vi "Main.vi"() -> ()   [LabVIEW 2017]
doc: "This Continuous Measurement sample project is based on the Queued Message Handler template.\n\nThe Event Handling Loop generates messages based on user interface actions.\n\nThe Message Handling Loop processes messages generated by the Event Handling Loop, or by other messages. There are also Acquisition and Logging message handling loop subVIs, and a chart updating loop."
uses:
  Settings/Settings.ctl
  Acquisition/Hardware Configuration.ctl
  Acquisition/Signal Type.ctl
  Settings/Terminal Configuration.ctl
  Settings/Range.ctl
  Settings/Coupling.ctl
  Settings/Sampling Clock Source.ctl
  Settings/Time Units.ctl
  Settings/Resolution.ctl
  Settings/Trigger Direction.ctl
  Settings/Trigger Source.ctl
  Settings/Quantity.ctl
  Logging/Logging Configuration.ctl
  controls/UI Data.ctl
  controls/UI State.ctl
  support/Active channels.vi
  support/Message Queue/Enqueue Message (Single).vi
  support/Message Queue/Enqueue Message (Array).vi
  <vilib>/Utility/error.llb/Error Cluster From Error Code.vi
  <vilib>/ErrorRing/Error Ring.xnode
  Acquisition/Acquisition.lvlib
  Logging/Logging.lvlib
  Settings/Settings.lvlib
  support/User Event - Stop/User Event - Stop.lvlib
  support/Message Queue/Message Queue.lvlib
  Settings/Settings Dialog.vi
panel:
  out "Actual sampling time [s]":dbl format="%^#_6e"
  out "Ch 2":bool
  out "Ch 1":bool
  in  "Min":dbl
  in  "Max":dbl
  out "Data":waveform(dbl)[](graph)
  in  "Settings":bool
  in  "Start":bool
  in  "Stop":bool
  out "Status":string
  in  "Exit":bool
  # "Limit values"
  # "Instrumentation Idea Fast Prototyping Lab"
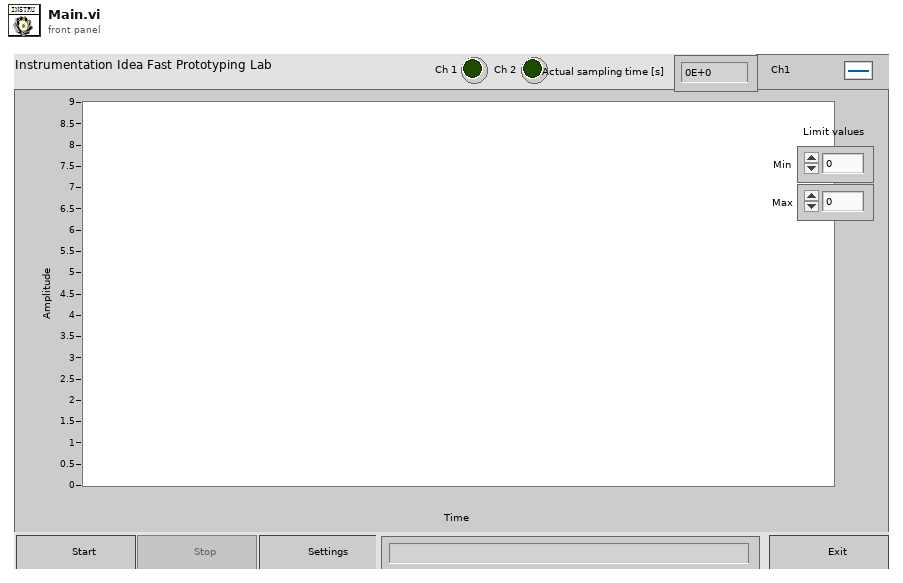
[diagram p1: front panel]
types:
  T1 = typedef "UI State.ctl" = enum16{"Idle", "Acquiring and Logging", "Waiting for Exit", "Waiting for Exit (Acq Stopped)", "Waiting for Exit (Log Stopped)", "Waiting for Stop", "Waiting for Stop (Acq Stopped)", "Waiting for Stop (Log Stopped)"}
  T2 = typedef "UI Data.ctl" = cluster{"Start Ref":refnum<vi>, "Stop Ref":refnum<vi>, "Settings Ref":refnum<vi>, "Exit Ref":refnum<vi>, "Status Ref":refnum<vi>, "Data Ref":refnum<vi>}
  T3 = typedef "Settings.lvlib/Settings.ctl" = cluster{"Hardware Configuration":T4, "Logging Configuration":T15}
  T4 = typedef "Acquisition.lvlib/Hardware Configuration.ctl" = cluster{"VISA resource name":refnum<visa-resource-name>, "DAQ Type":T5, "Channel 1":cluster{"Acquiring":bool, "Enabled":bool, "Terminal configuration":T6, "Range":T7, "Coupling":T8}, "Channel 2":cluster{"Acquiring":bool, "Enabled":bool, "Terminal configuration":T6, "Range":T7, "Coupling":T8}, "Timing":cluster{"Sample Time [Time Units]":u32, "Actual Sample Time [s]":dbl, "Samples per Iteration":u32, "Sample Clock Source":T9, "Time Units":T10, "t0":timestamp, "Baud rate":u32}, "PS Parameters":cluster{"PS handle":i16, "PS Max_adc":i16, "PS Enabled Array":i16[], "PS Device Info":cluster{"Driver Version":string, "USB Version":string, "Hardware":string, "Variant":string, "Batch and Serial":string, "Cal Date":string, "Kernel Version":string, "Digital HW Version":string, "Analogue HW Version":string, "Firmware 1":string, "Firmware 2":string, "MSO":bool, "Number of Channels":i16}, "Channel 1 Buffer":refnum<data-value>, "Channel 2 Buffer":refnum<data-value>, "Resolution":T11, "USB Power":bool}, "Trigger":cluster{"Direction":T12, "Threshold [V]":dbl, "Enabled":bool, "Trigger Source":T13}, "Keithley Parameters":cluster{"Previous End / Current Start":i32, "Quantity":T14}}
  T5 = typedef "Acquisition.lvlib/Signal Type.ctl" = u16
  T6 = typedef "Settings.lvlib/Terminal Configuration.ctl" = u16
  T7 = typedef "Settings.lvlib/Range.ctl" = u16
  T8 = typedef "Settings.lvlib/Coupling.ctl" = i16
  T9 = typedef "Settings.lvlib/Sampling Clock Source.ctl" = u16
  T10 = typedef "Settings.lvlib/Time Units.ctl" = u32
  T11 = typedef "Settings.lvlib/Resolution.ctl" = i32
  T12 = typedef "Settings.lvlib/Trigger Direction.ctl" = u16
  T13 = typedef "Settings.lvlib/Trigger Source.ctl" = u16
  T14 = typedef "Settings.lvlib/Quantity.ctl" = u16
  T15 = typedef "Logging.lvlib/Logging Configuration.ctl" = cluster{"Log File Base Path":path, "TDMS File Reference":refnum<k34>, "Enabled":bool, "Disk cache size":u64}
  T16 = typedef "Message Queue.lvlib/All Message Queues.ctl" = cluster{"UI":refnum<queue>, "Acquisition":refnum<queue>, "Logging":refnum<queue>}
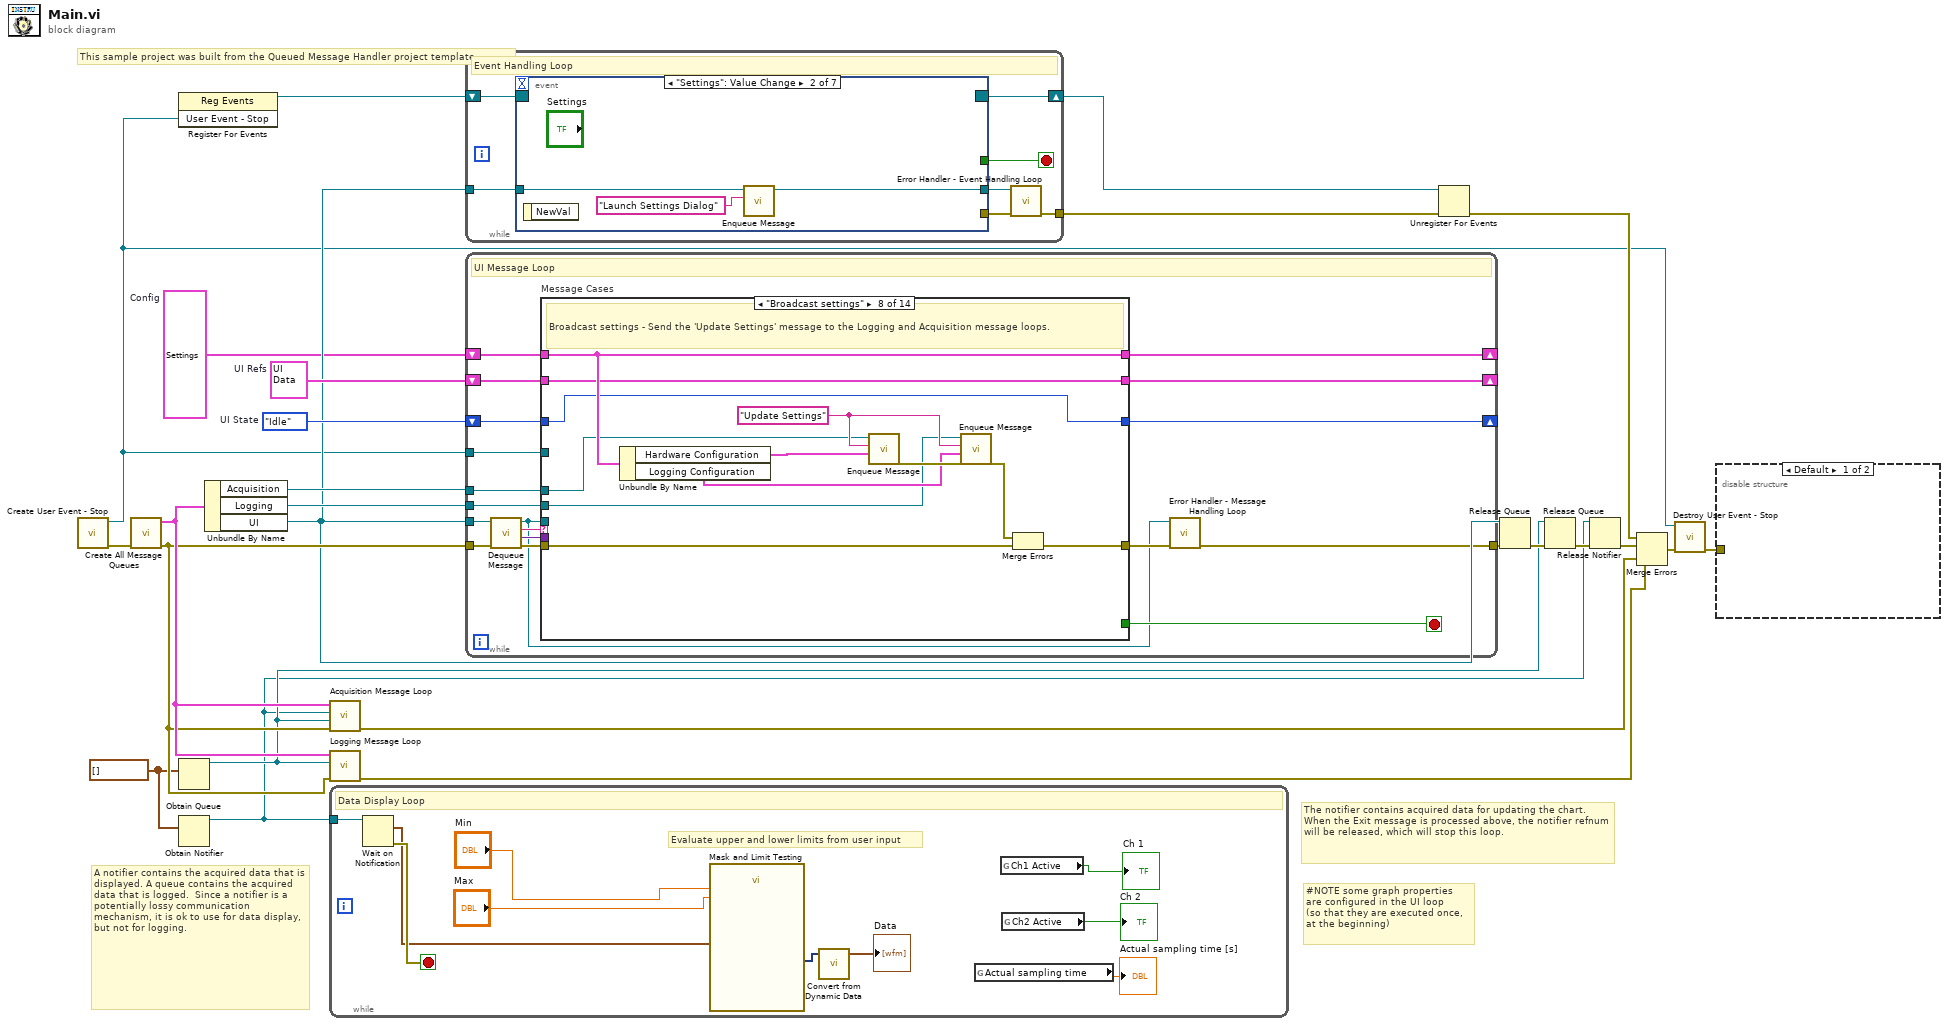
[diagram p0: block diagram]
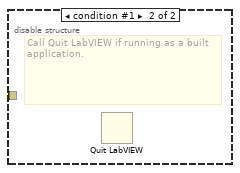
[diagram p2: hidden frame]
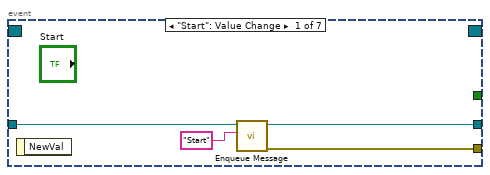
[diagram p3: hidden frame]
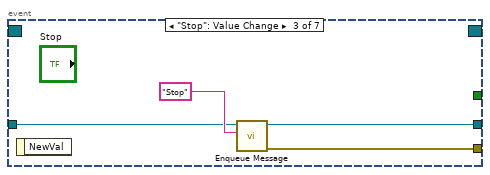
[diagram p4: hidden frame]
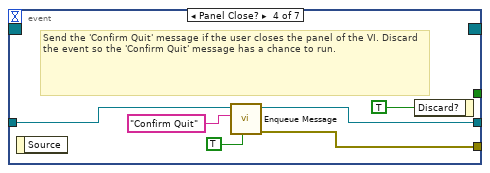
[diagram p5: hidden frame]
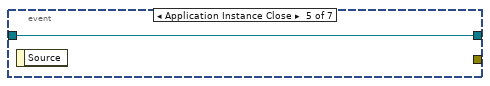
[diagram p6: hidden frame]
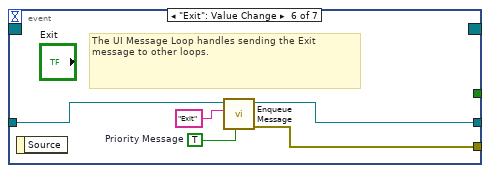
[diagram p7: hidden frame]
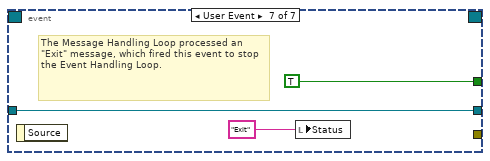
[diagram p8: hidden frame]
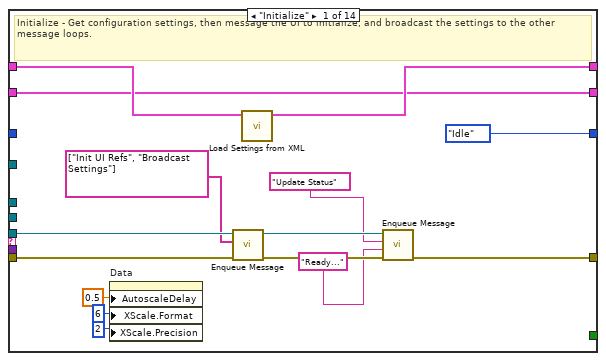
[diagram p9: hidden frame]
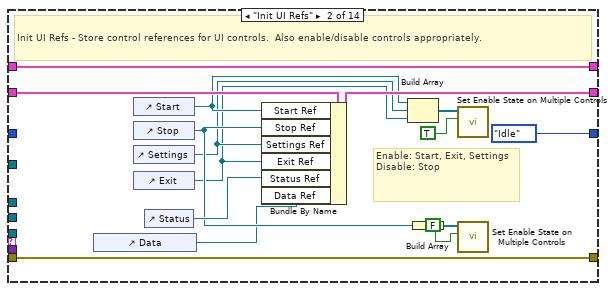
[diagram p10: hidden frame]
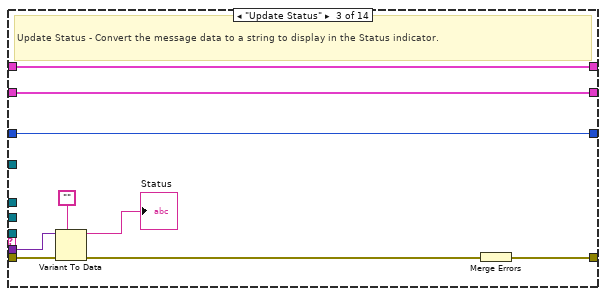
[diagram p11: hidden frame]
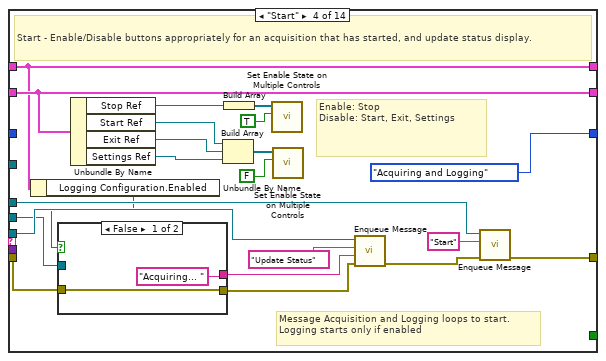
[diagram p12: hidden frame]
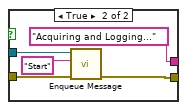
[diagram p13: hidden frame]
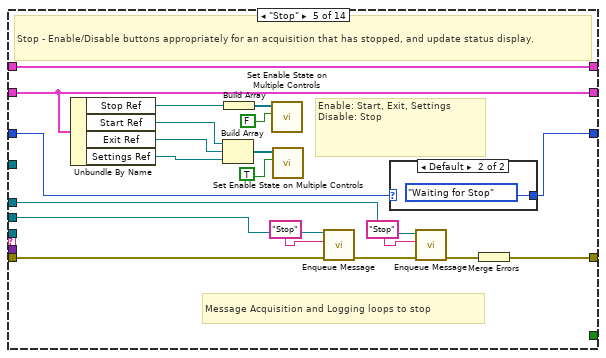
[diagram p14: hidden frame]
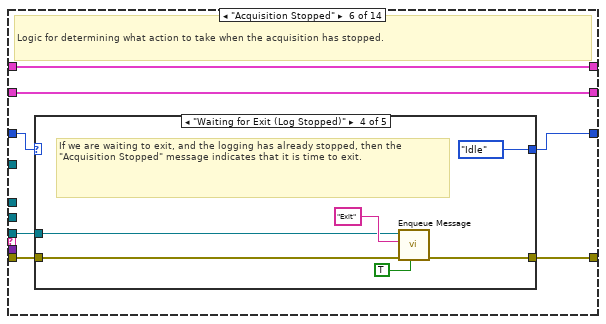
[diagram p16: hidden frame]
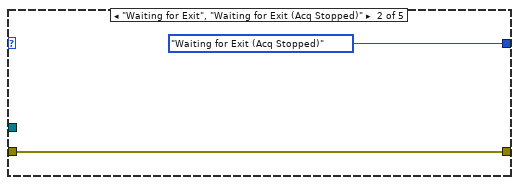
[diagram p18: hidden frame]
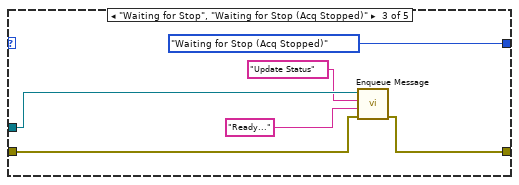
[diagram p19: hidden frame]
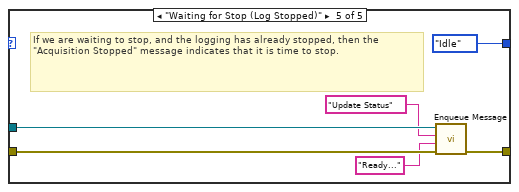
[diagram p20: hidden frame]
diagram:
  w13 = UI_State."Idle"  # UI State
  w4 = waveform(dbl)[] []
  w16 = T2 {"Start Ref"=refnum, "Stop Ref"=refnum, "Settings Ref"=refnum, "Exit Ref"=refnum, "Status Ref"=refnum, "Data Ref"=refnum}  # UI Refs
  w1 = T3 {"Hardware Configuration"={"VISA resource name"="", "DAQ Type"=0, "Channel 1"={"Acquiring"=FALSE, "Enabled"=FALSE, "Terminal configuration"=0, "Range"=32767, "Coupling"=0}, "Channel 2"={"Acquiring"=FALSE, "Enabled"=FALSE, "Terminal configuration"=0, "Range"=0, "Coupling"=0}, "Timing"={"Sample Time [Time Units]"=0, "Actual Sample Time [s]"=0.0, "Samples per Iteration"=0, "Sample Clock Source"=0, "Time Units"=0, "t0"=timestamp(0 s since 1904-01-01), "Baud rate"=0}, "PS Parameters"={"PS handle"=0, "PS Max_adc"=32767, "PS Enabled Array"=[], "PS Device Info"={"Driver Version"="", "USB Version"="", "Hardware"="", "Variant"="", "Batch and Serial"="", "Cal Date"="", "Kernel Version"="", "Digital HW Version"="", "Analogue HW Version"="", "Firmware 1"="", "Firmware 2"="", "MSO"=FALSE, "Number of Channels"=0}, "Channel 1 Buffer"=refnum, "Channel 2 Buffer"=refnum, "Resolution"=0, "USB Power"=FALSE}, "Trigger"={"Direction"=0, "Threshold [V]"=0.0, "Enabled"=FALSE, "Trigger Source"=0}, "Keithley Parameters"={"Previous End / Current Start"=0, "Quantity"=0}}, "Logging Configuration"={"Log File Base Path"=path "", "TDMS File Reference"=refnum, "Enabled"=FALSE, "Disk cache size"=0}}  # Config
  # "#NOTE some graph properties\nare configured in the UI loop \n(so that they are executed once,\nat the beginning)"
  # "This sample project was built from the Queued Message Handler project template."
  # "A notifier contains the acquired data that is displayed. A queue contains the acquired data that is logged.  Since a notifier is a potentially lossy communication mechanism, it is ok to use for data display, but not for logging."
  # "The notifier contains acquired data for updating the chart. When the Exit message is processed above, the notifier refnum will be released, which will stop this loop."
  n1 = call "Create User Event - Stop.vi"() -> ("error out"=w22:errorcluster, "User Event - Stop"=w2:refnum<user-event>)  [unwired: 10 in]
  n2 = call "Create All Message Queues.vi"("error in (no error)"=w22) -> ("error out"=w19:errorcluster, "Message Queues out"=w21:T16)  [unwired: 9 in]
  n3 = register-events(w2) -> (reference out=w3:refnum<event-registration>)  [unwired: 2 in, 1 out]
  n4 = Obtain Queue(element data type=w4) -> (queue out=w6:refnum<queue>)  [unwired: 4 in, 2 out]
  n5 = Obtain Notifier(notification data type=w4) -> (notifier out=w5:refnum<notifier>)  [unwired: 3 in, 2 out]
  n6 = Unbundle By Name(w21) -> ("Acquisition"=w15:refnum<queue>, "Logging"=w14:refnum<queue>, "UI"=w11:refnum<queue>)
  n7 = call "Acquisition Message Loop.vi"("error in (no error)"=w19, "Data Queue"=w6, "Data Notifier"=w5, "Message Queues"=w21) -> ("error out"=w23:errorcluster)  [unwired: 7 in]
  n8 = call "Logging Message Loop.vi"("error in (no error)"=w19, "Data Queue"=w6, "Message Queues"=w21) -> ("error out"=w20:errorcluster)  [unwired: 8 in]
  n9 = while "Data Display Loop" {
    tunnel: w5 -> [w35]
    stop <- w34 stop-if-true
    # "Evaluate upper and lower limits from user input"
    # "Data Display Loop"
    n10 = Wait on Notification(notifier=w35) -> (notification=w29:waveform(dbl)[], error out=w34:errorcluster)  [unwired: 3 in, 2 out]
    n11 = call "Mask and Limit Testing"("Lower Constant"="Min", "Upper Constant"="Max", "Signals"=w29) -> ("Tested Signals"=w33:dynamicdata)  [unwired: 5 in, 3 out]
    n12 = call "Convert from Dynamic Data"("Dynamic Data Type"=w33) -> ("Array of Waveform"=→"Data":waveform(dbl)[])  [unwired: 3 in]
    n13 = global read "Active channels.vi" "Actual sampling time"() -> (→"Actual sampling time [s]":dbl)
    n14 = global read "Active channels.vi" "Ch1 Active"() -> (→"Ch 1":bool)
    n15 = global read "Active channels.vi" "Ch2 Active"() -> (→"Ch 2":bool)
  }
  n16 = while {
    tunnel: w11 -> [w41]
    tunnel: [w38] -> w24
    shift-right: [w40] -> w17
    shift-left: w3 -> [w42]
    stop <- w39 stop-if-true
    # "Event Handling Loop"
    n17 = event shown="[1] \"Settings\": Value Change" {
      selector: w42 -> [_ _ _ _ _ _ _]
      dyn-events: [_ _ _ _ _ _ _] -> w40
      timeout: _ -> [_ _ _ _ _ _ _]
      tunnel: [_ _ _ _ _ _ TRUE ("Discard?")] -> w39
      tunnel: w41 -> [w46 w48 w52 w57 w60 w62 w66]
      tunnel: [w44 _ w51 w55 _ w65 _] -> w37
      tunnel: [w43 w47 w50 w56 w60 w61 w66] -> w36
      event "Start": Value Change {
        n18 = event-data() -> ()  [unwired: 1 in, 1 out]
        n19 = call-poly "Enqueue Message.vi"("Message"="Start", "Message Queue"=w46) -> ("error out"=w44:errorcluster, "dup Message Queue"=w43:refnum<queue>)  [unwired: 8 in]
      }
      event "Settings": Value Change {
        n20 = event-data() -> ()  [unwired: 1 in, 1 out]
        n21 = call-poly "Enqueue Message.vi"("Message"="Launch Settings Dialog", "Message Queue"=w48) -> ("dup Message Queue"=w47:refnum<queue>)  [unwired: 8 in, 1 out]
      }
      event "Stop": Value Change {
        n22 = event-data() -> ()  [unwired: 1 in, 1 out]
        n23 = call-poly "Enqueue Message.vi"("Message"="Stop", "Message Queue"=w52) -> ("error out"=w51:errorcluster, "dup Message Queue"=w50:refnum<queue>)  [unwired: 8 in]
      }
      event Panel Close? {
        # "Send the 'Confirm Quit' message if the user closes the panel of the VI. Discard the event so the 'Confirm Quit' message has a chance to run."
        n24 = event-data() -> ()  [unwired: 1 in, 1 out]
        n25 = call-poly "Enqueue Message.vi"("Priority Message? (F)"=TRUE, "Message"="Confirm Quit", "Message Queue"=w57) -> ("error out"=w55:errorcluster, "dup Message Queue"=w56:refnum<queue>)  [unwired: 7 in]
        n26 = event-data("Discard?"=TRUE) -> ()  [unwired: 1 in, 1 out]
      }
      event Application Instance Close {
        n27 = event-data() -> ()  [unwired: 1 in, 1 out]
      }
      event "Exit": Value Change {
        w63 = TRUE  # Priority Message
        # "The UI Message Loop handles sending the Exit message to other loops."
        n28 = event-data() -> ()  [unwired: 1 in, 1 out]
        n29 = call-poly "Enqueue Message.vi"("Priority Message? (F)"=w63, "Message"="Exit", "Message Queue"=w62) -> ("error out"=w65:errorcluster, "dup Message Queue"=w61:refnum<queue>)  [unwired: 7 in]
      }
      event User Event {
        # "The Message Handling Loop processed an \"Exit\" message, which fired this event to stop the Event Handling Loop."
        n30 = event-data() -> ()  [unwired: 1 in, 1 out]
        n31 = local write "Status"("Exit" ("Exit String")) -> ()
      }
    }
    n32 = call "Error Handler - Event Handling Loop.vi"("error in (no error)"=w37, "Message Queue"=w36) -> ("dup error in"=w38:errorcluster)  [unwired: 8 in, 1 out]
  }
  n33 = while {
    tunnel: w11 -> [w80]
    tunnel: w2 -> [w85]
    shift-right: [w70] -> _
    shift-left: w1 -> [w69]
    shift-right: [w78] -> _
    shift-left: w16 -> [w79]
    tunnel: w15 -> [w77]
    tunnel: w14 -> [w76]
    shift-right: [w71] -> _
    shift-left: w13 -> [w72]
    tunnel: w19 -> [w84]
    tunnel: [w75] -> w25
    stop <- w86 stop-if-true
    # "UI Message Loop"
    n34 = call "Dequeue Message.vi"("error in (no error)"=w84, "Message Queue"=w80) -> ("error out"=w83:errorcluster, "Message Data"=w81:variant, "Message"=w82:string, "dup Message Queue"=w73:refnum<queue>)  [unwired: 6 in]
    n35 = case "Message Cases" shown="\"Broadcast settings\"" w82 {
      selector: w82 -> [_ _ _ _ _ _ _ _ _ _ _ _ _ w316]
      tunnel: w73 -> [w93 _ _ w147 _ w179 w208 _ w248 _ w269 _ _ _]
      tunnel: w83 -> [w92 w116 w124 w129 w173 w180 w209 w236 w250 w257 w268 w297 w314 _]
      tunnel: [w97 w116 w125 w134 w174 w177 w206 w242 w243 w260 w267 w307 w313 w315] -> w74
      tunnel: [_ _ _ _ _ _ _ _ _ _ _ TRUE _ _] -> w86
      tunnel: w81 -> [_ _ w123 _ _ _ _ _ _ w261 _ w295 _ _]
      tunnel: w85 -> [_ _ _ _ _ _ _ _ _ _ _ w308 _ _]
      tunnel: [w100 w115 w119 w130 w172 w183 w212 w240 w247 w265 w272 w306 w312 w319] -> w70
      tunnel: w69 -> [w101 w115 w119 w130 w172 w183 w212 w240 w251 w265 w272 w306 w312 w319]
      tunnel: w79 -> [w94 w114 w118 w144 w171 w182 w211 w234 w245 w264 w271 w305 w311 w318]
      tunnel: [w94 w112 w118 w144 w171 w182 w211 w234 w245 w264 w271 w305 w311 w318] -> w78
      tunnel: w77 -> [_ _ _ w133 w158 _ _ w233 _ _ _ w304 _ _]
      tunnel: w76 -> [_ _ _ w135 w161 _ _ w232 _ _ _ w303 _ _]
      tunnel: w72 -> [_ _ w117 _ w155 w181 w210 w231 w244 w259 w270 _ w310 w317]
      tunnel: [UI_State."Idle" ("UI State") UI_State."Idle" ("UI State") w117 UI_State."Acquiring and Logging" ("UI State") w156 w178 w207 w231 w244 w259 w266 UI_State."Idle" ("UI State") w310 w317] -> w71
      frame "Initialize" {
        # "Initialize - Get configuration settings, then message the UI to initialize, and broadcast the settings to the other message loops."
        n36 = property on="Data" class="WFChart (strict)"("AutoscaleDelay"=sgl 0.5 ("Autoscale Delay"), "XScale.Format"=u8 6 ("X Scale.Display Format:Format"), "XScale.Precision"=u8 2 ("X Scale.Display Format:Precision")) -> ()  [unwired: 2 in, 2 out]
        n37 = call-poly "Enqueue Message.vi"("error in (no error)"=w92, "Message Array"=string[] ["Init UI Refs", "Broadcast Settings"], "Message Queue"=w93) -> ("error out"=w99:errorcluster, "dup Message Queue"=w98:refnum<queue>)  [unwired: 7 in]
        n38 = call "Load Settings from XML.vi"("Settings in"=w101) -> ("Settings out"=w100:T3)  [unwired: 9 in, 1 out]
        n39 = call-poly "Enqueue Message.vi"("error in (no error)"=w99, "Message Data"="Ready..." ("Ready..."), "Message"="Update Status", "Message Queue"=w98) -> ("error out"=w97:errorcluster)  [unwired: 6 in, 1 out]
      }
      frame "Init UI Refs" {
        # "Enable: Start, Exit, Settings\nDisable: Stop"
        # "Init UI Refs - Store control references for UI controls.  Also enable/disable controls appropriately."
        n40 = control-ref of="Data"() -> (w102:refnum<vi>)
        n41 = control-ref of="Start"() -> (w106:refnum<vi>)
        n42 = control-ref of="Stop"() -> (w107:refnum<vi>)
        n43 = control-ref of="Settings"() -> (w105:refnum<vi>)
        n44 = control-ref of="Exit"() -> (w104:refnum<vi>)
        n45 = control-ref of="Status"() -> (w113:refnum<vi>)
        n46 = Bundle By Name(cluster=w114, "Start Ref"=w106, "Stop Ref"=w107, "Settings Ref"=w105, "Exit Ref"=w104, "Status Ref"=w113, "Data Ref"=w102) -> (w112:T2)
        n47 = Build Array(w106, w105, w104) -> (w110:refnum<vi>[])
        n48 = Build Array(w107) -> (w109:refnum<vi>[])
        n49 = call "Set Enable State on Multiple Controls.vi"("Enable?"=TRUE, "Controls"=w110) -> ()  [unwired: 10 in]
        n50 = call "Set Enable State on Multiple Controls.vi"("Enable?"=FALSE, "Controls"=w109) -> ()  [unwired: 10 in]
      }
      frame "Update Status" {
        # "Update Status - Convert the message data to a string to display in the Status indicator."
        n51 = Variant To Data(error in=w124, type="", Variant=w123) -> (data=→"Status":string, error out=w121:errorcluster)
        n52 = Merge Errors(w121) -> (w125:errorcluster)
      }
      frame "Start" {
        # "Message Acquisition and Logging loops to start.\nLogging starts only if enabled"
        # "Enable: Stop\nDisable: Start, Exit, Settings"
        # "Start - Enable/Disable buttons appropriately for an acquisition that has started, and update status display."
        n53 = Unbundle By Name(w130) -> ("Logging Configuration.Enabled"=w126:bool)
        n54 = case shown="False" w126 {
          tunnel: ["Acquiring... " ("Acquiring and Logging...") "Acquiring and Logging..." ("Acquiring and Logging...")] -> w146
          tunnel: w135 -> [_ w153]
          tunnel: w129 -> [w148 w151]
          tunnel: [w148 w150] -> w128
          frame False {
          }
          frame True {
            n55 = call-poly "Enqueue Message.vi"("error in (no error)"=w151, "Message"="Start", "Message Queue"=w153) -> ("error out"=w150:errorcluster)  [unwired: 7 in, 1 out]
          }
        }
        n56 = Unbundle By Name(w144) -> ("Stop Ref"=w139:refnum<vi>, "Start Ref"=w138:refnum<vi>, "Exit Ref"=w137:refnum<vi>, "Settings Ref"=w136:refnum<vi>)
        n57 = Build Array(w138, w137, w136) -> (w142:refnum<vi>[])
        n58 = Build Array(w139) -> (w141:refnum<vi>[])
        n59 = call "Set Enable State on Multiple Controls.vi"("Enable?"=TRUE, "Controls"=w141) -> ()  [unwired: 10 in]
        n60 = call "Set Enable State on Multiple Controls.vi"("Enable?"=FALSE, "Controls"=w142) -> ()  [unwired: 10 in]
        n61 = call-poly "Enqueue Message.vi"("error in (no error)"=w128, "Message Data"=w146, "Message"="Update Status", "Message Queue"=w147) -> ("error out"=w127:errorcluster)  [unwired: 6 in, 1 out]
        n62 = call-poly "Enqueue Message.vi"("error in (no error)"=w127, "Message"="Start", "Message Queue"=w133) -> ("error out"=w134:errorcluster)  [unwired: 7 in, 1 out]
      }
      frame "Stop" {
        # "Message Acquisition and Logging loops to stop"
        # "Enable: Start, Exit, Settings\nDisable: Stop"
        # "Stop - Enable/Disable buttons appropriately for an acquisition that has stopped, and update status display."
        n63 = Unbundle By Name(w171) -> ("Stop Ref"=w166:refnum<vi>, "Start Ref"=w165:refnum<vi>, "Exit Ref"=w164:refnum<vi>, "Settings Ref"=w163:refnum<vi>)
        n64 = Build Array(w165, w164, w163) -> (w169:refnum<vi>[])
        n65 = Build Array(w166) -> (w168:refnum<vi>[])
        n66 = call "Set Enable State on Multiple Controls.vi"("Enable?"=FALSE, "Controls"=w168) -> ()  [unwired: 10 in]
        n67 = call "Set Enable State on Multiple Controls.vi"("Enable?"=TRUE, "Controls"=w169) -> ()  [unwired: 10 in]
        n68 = call-poly "Enqueue Message.vi"("error in (no error)"=w173, "Message"="Stop", "Message Queue"=w161) -> ("error out"=w160:errorcluster)  [unwired: 7 in, 1 out]
        n69 = case shown="Default" w155 {
          selector: w155 -> [w175 _]
          tunnel: [w175 UI_State."Waiting for Stop" ("UI State")] -> w156
          frame "Waiting for Exit" {
          }
          frame Default {
          }
        }
        n70 = call-poly "Enqueue Message.vi"("error in (no error)"=w160, "Message"="Stop", "Message Queue"=w158) -> ("error out"=w159:errorcluster)  [unwired: 7 in, 1 out]
        n71 = Merge Errors(w159) -> (w174:errorcluster)
      }
      frame "Acquisition Stopped" {
        # "Logic for determining what action to take when the acquisition has stopped."
        n72 = case shown="\"Waiting for Exit (Log Stopped)\"" w181 {
          selector: w181 -> [w185 _ _ _ _]
          tunnel: w180 -> [w184 w187 w189 w194 w205]
          tunnel: w179 -> [_ _ w192 w195 w202]
          tunnel: [w185 UI_State."Waiting for Exit (Acq Stopped)" ("UI State") UI_State."Waiting for Stop (Acq Stopped)" ("UI State") UI_State."Idle" ("UI State") UI_State."Idle" ("UI State")] -> w178
          tunnel: [w184 w187 w188 w199 w203] -> w177
          frame Default {
          }
          frame "Waiting for Exit", "Waiting for Exit (Acq Stopped)" {
          }
          frame "Waiting for Stop", "Waiting for Stop (Acq Stopped)" {
            n73 = call-poly "Enqueue Message.vi"("error in (no error)"=w189, "Message Data"="Ready..." ("Ready..."), "Message"="Update Status", "Message Queue"=w192) -> ("error out"=w188:errorcluster)  [unwired: 6 in, 1 out]
          }
          frame "Waiting for Exit (Log Stopped)" {
            # "If we are waiting to exit, and the logging has already stopped, then the \"Acquisition Stopped\" message indicates that it is time to exit."
            n74 = call-poly "Enqueue Message.vi"("Priority Message? (F)"=TRUE, "error in (no error)"=w194, "Message"="Exit", "Message Queue"=w195) -> ("error out"=w199:errorcluster)  [unwired: 6 in, 1 out]
          }
          frame "Waiting for Stop (Log Stopped)" {
            # "If we are waiting to stop, and the logging has already stopped, then the \"Acquisition Stopped\" message indicates that it is time to stop."
            n75 = call-poly "Enqueue Message.vi"("error in (no error)"=w205, "Message Data"="Ready..." ("Ready..."), "Message"="Update Status", "Message Queue"=w202) -> ("error out"=w203:errorcluster)  [unwired: 6 in, 1 out]
          }
        }
      }
      frame "Logging Stopped" {
        # "Logic for determining what action to take when the logging has stopped."
        n76 = case shown="\"Waiting for Stop (Acq Stopped)\"" w210 {
          selector: w210 -> [w214 _ _ _ _]
          tunnel: w209 -> [w213 w216 w218 w224 w227]
          tunnel: w208 -> [_ _ _ w222 w226]
          tunnel: [w214 UI_State."Waiting for Exit (Log Stopped)" ("UI State") UI_State."Waiting for Stop (Log Stopped)" ("UI State") UI_State."Idle" ("UI State") UI_State."Idle" ("UI State")] -> w207
          tunnel: [w213 w216 w218 w223 w225] -> w206
          frame Default {
          }
          frame "Waiting for Exit", "Waiting for Exit (Log Stopped)" {
          }
          frame "Waiting for Stop", "Waiting for Stop (Log Stopped)" {
          }
          frame "Waiting for Exit (Acq Stopped)" {
            # "If we are waiting to exit, and the acquisition has already stopped, then the \"Logging Stopped\" message indicates that it is time to exit."
            n77 = call-poly "Enqueue Message.vi"("Priority Message? (F)"=TRUE, "error in (no error)"=w224, "Message"="Exit", "Message Queue"=w222) -> ("error out"=w223:errorcluster)  [unwired: 6 in, 1 out]
          }
          frame "Waiting for Stop (Acq Stopped)" {
            # "If we are waiting to stop, and the acquisition has already stopped, then the \"Logging Stopped\" message indicates that it is time to stop."
            n78 = call-poly "Enqueue Message.vi"("error in (no error)"=w227, "Message Data"="Ready..." ("Ready..."), "Message"="Update Status", "Message Queue"=w226) -> ("error out"=w225:errorcluster)  [unwired: 6 in, 1 out]
          }
        }
      }
      frame "Broadcast settings" {
        w235 = "Update Settings" ("Message")
        # "Broadcast settings - Send the 'Update Settings' message to the Logging and Acquisition message loops."
        n79 = Unbundle By Name(w240) -> ("Hardware Configuration"=w239:T4, "Logging Configuration"=w238:T15)
        n80 = call-poly "Enqueue Message.vi"("Message Data"=w239, "Message"=w235, "Message Queue"=w233) -> ("error out"=w241:errorcluster)  [unwired: 7 in, 1 out]
        n81 = call-poly "Enqueue Message.vi"("error in (no error)"=w241, "Message Data"=w238, "Message"=w235, "Message Queue"=w232) -> ("error out"=w237:errorcluster)  [unwired: 6 in, 1 out]
        n82 = Merge Errors(w237, w236) -> (w242:errorcluster)
      }
      frame "Launch Settings Dialog" {
        # "Launch Settings Dialog - Launch the Settings Dialog when the user clicks the 'Settings' button."
        n83 = call-by-ref "?"("error in (no error)"=w250, "Settings in"=w251) -> ("error out"=w246:errorcluster, "Cancelled?"=w249:bool, "Settings out"=w247:T3)  [unwired: 8 in, 3 out]
        n84 = case shown="False" w249 {
          tunnel: w248 -> [w255 _]
          tunnel: w246 -> [w254 w256]
          tunnel: [w253 w256] -> w243
          frame False {
            n85 = call-poly "Enqueue Message.vi"("error in (no error)"=w254, "Message"="Broadcast Settings", "Message Queue"=w255) -> ("error out"=w253:errorcluster)  [unwired: 7 in, 1 out]
          }
          frame True {
          }
        }
      }
      frame "Error" {
        # "Error - Display an error dialog. This message is sent by the \"Error Handler\" VIs at the end of other loops in this application."
        n86 = Variant To Data(error in=w257, type=errorcluster {"status"=FALSE, "code"=0, "source"=""} ("error constant"), Variant=w261) -> (data=w258:errorcluster, error out=w262:errorcluster)
        n87 = call <vilib>:"Simple Error Handler.vi"("error in (no error)"=w258) -> ()  [unwired: 4 in, 5 out]
        n88 = Merge Errors(w262) -> (w260:errorcluster)
      }
      frame "Confirm Quit" {
        # "Confirm Quit - Message that can confirm whether or not the user wants to exit the application."
        n89 = case shown="Default" w270 {
          tunnel: w269 -> [w278 w282]
          tunnel: w268 -> [w277 w281]
          tunnel: [w276 w280] -> w267
          tunnel: [UI_State."Idle" ("UI State") w279] -> w266
          frame Default {
            # "If 'Confirm Quit' comes in while the system is idle, there is no need for a confirmation message."
            n90 = call-poly "Enqueue Message.vi"("Priority Message? (F)"=TRUE, "error in (no error)"=w277, "Message"="Exit", "Message Queue"=w278) -> ("error out"=w276:errorcluster)  [unwired: 6 in, 1 out]
          }
          frame "Acquiring and Logging" {
            n91 = Two Button Dialog(message="Are you sure you want to quit while the acquisition is running?" ("Confirm Quit Message"), 1:"No" ("No"), 2:"Yes" ("Yes")) -> (T button?=w283:bool)
            n92 = case shown="True" w283 {
              tunnel: w282 -> [_ w292]
              tunnel: w281 -> [w288 w293]
              tunnel: [w288 w291] -> w280
              tunnel: [UI_State."Acquiring and Logging" ("UI State") UI_State."Waiting for Exit" ("UI State")] -> w279
              frame False {
                # "User did not want to quit."
              }
              frame True {
                n93 = call-poly "Enqueue Message.vi"("error in (no error)"=w293, "Message"="Stop", "Message Queue"=w292) -> ("error out"=w291:errorcluster)  [unwired: 7 in, 1 out]
              }
            }
          }
        }
      }
      frame "Exit" {
        w299 = TRUE ("Priority Message? (F)")
        w300 = "Exit" ("Message")
        # "Popup an error dialog if 'Exit' was called as a result of an error."
        # "Stop the VI"
        # "Exit - Send Exit messages to the Acquisition and Logging loops, and fire the user event to stop the Event Handling Loop."
        n94 = Variant To Data(type=errorcluster {"status"=FALSE, "code"=0, "source"=""} ("error constant"), Variant=w295) -> (data=w294:errorcluster)  [unwired: 1 in, 1 out]
        n95 = call <vilib>:"Simple Error Handler.vi"("error in (no error)"=w294) -> ()  [unwired: 4 in, 5 out]
        n96 = call-poly "Enqueue Message.vi"("Priority Message? (F)"=w299, "error in (no error)"=w297, "Message"=w300, "Message Queue"=w304) -> ("error out"=w301:errorcluster)  [unwired: 6 in, 1 out]
        n97 = call-poly "Enqueue Message.vi"("Priority Message? (F)"=w299, "error in (no error)"=w301, "Message"=w300, "Message Queue"=w303) -> ("error out"=w298:errorcluster)  [unwired: 6 in, 1 out]
        n98 = call "Fire User Event - Stop.vi"("error in (no error)"=w298, "User Event - Stop"=w308) -> ("error out"=w307:errorcluster)  [unwired: 9 in]
      }
      frame "---Copy This Frame---" {
        # "Duplicate this frame when creating new messages.  Change this comment in the duplicated frame to describe this message."
        n99 = Merge Errors(w314) -> (w313:errorcluster)
      }
      frame Default {
        # "'Default' case only runs if there is a message that isn't defined in any of the other cases.  Output a programming error."
        n100 = xnode "Error Ring"("parameter 0"=w316) -> ("error out"=w315:errorcluster)
      }
    }
    n101 = call "Error Handler - Message Handling Loop.vi"("error in (no error)"=w74, "Message Queue"=w73) -> ("dup error in"=w75:errorcluster)  [unwired: 8 in, 1 out]
  }
  n102 = Unregister For Events(event registration refnum=w17, error in=w24) -> (error out=w18:errorcluster)
  n103 = Release Queue(queue=w11, error in (no error)=w25) -> (error out=w9:errorcluster)  [unwired: 1 in, 2 out]
  n104 = Release Queue(queue=w6, error in (no error)=w9) -> (error out=w8:errorcluster)  [unwired: 1 in, 2 out]
  n105 = Release Notifier(notifier=w5, error in (no error)=w8) -> (error out=w7:errorcluster)  [unwired: 1 in, 2 out]
  n106 = Merge Errors(w18, w7, w23, w20) -> (w12:errorcluster)
  n107 = call "Destroy User Event - Stop.vi"("error in (no error)"=w12, "User Event - Stop"=w2) -> ("error out"=w10:errorcluster)  [unwired: 9 in]
  n108 = disable-structure shown="Default" {
    disable-tunnel: w10 -> [_ _]
    frame condition #0 (active) {
    }
    frame condition #1 {
      # "Call Quit LabVIEW if running as a built application."
      n109 = Quit LabVIEW() -> ()  [unwired: 1 in]
    }
  }
